vi "LVClass_Camera asynchroneImageReady.vi"(0 "Camera in":refnum<class "Camera.lvclass">, 11 "error in (no error)":errorcluster) -> (4 "Camera out":refnum<class "Camera.lvclass">, 6 "ready":bool, 15 "error out":errorcluster)   [LabVIEW 2020, in "Camera.lvclass"]
doc: "Indicates if a new image is available.\n\n<B>CameraIn</B> : Camera object.\n<B>CameraOut</B> : Camera object.\n<B>is_ready</B> : image availability in asynchronous image synchronization mode."
uses:
  Camera.lvclass
  Camera.lvclass/Camera.ctl
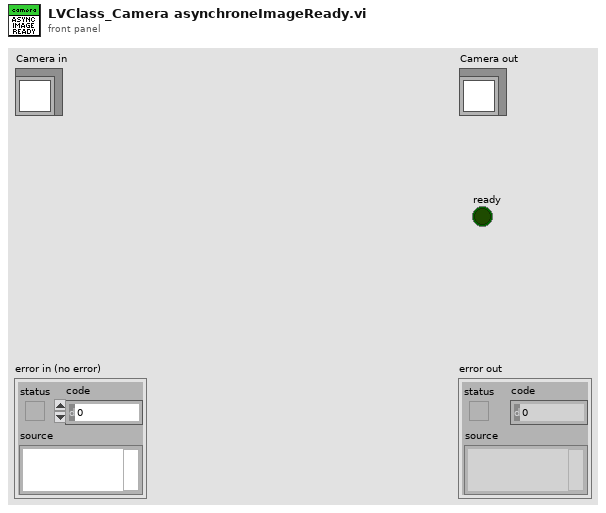
[diagram p1: front panel]
types:
  T1 = typedef "ClassID.ctl" = i64
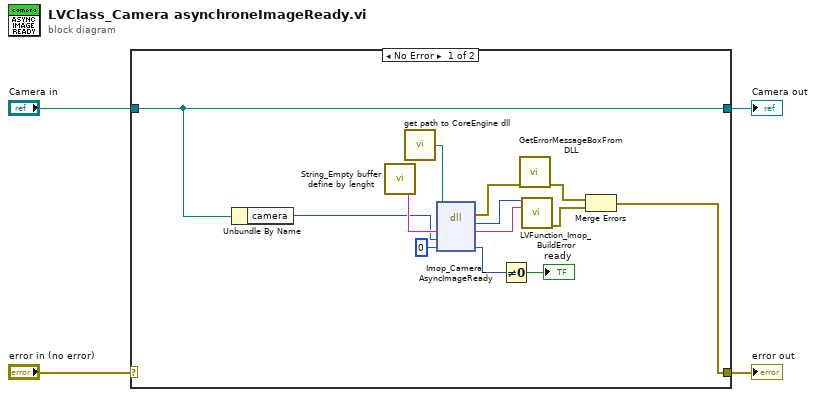
[diagram p0: block diagram]
diagram:
  n1 = case shown="No Error" "error in (no error)" {
    selector: "error in (no error)" -> [_ w19]
    tunnel: [w5 w19] -> w3
    tunnel: [w9 w18] -> w1
    tunnel: "Camera in" -> [w9 w18]
    frame No Error {
      n2 = Unbundle By Name(w9) -> ("camera"=w8:T1)
      n3 = call "String_Empty buffer define by lenght.vi"() -> ("Empty buffer"=w17:string)  [unwired: 1 in]
      n4 = call "get path to CoreEngine dll.vi"() -> ("path to c_interface_vc100.dll"=w14:path)  [unwired: 12 in, 3 out]
      n5 = dll-call lib="D:/SOFTware/HASO_v3/SVN_trunk/ImOpCoreEngine4_LV2011/DLLs/ImopEngine4_vc100.dll" fn="Imop_Camera_AsyncImageReady"(path in=w14, "message"=w17, "camera"=w8, "ready"=u8 0) -> (error out=w13:errorcluster, "return type"=w16:i32, "message"=w15:string, "ready"=w11:u8)  [unwired: 3 in, 1 out]
      n6 = Not Equal To 0?(x=w11) -> (x != 0?=→"ready":bool)
      n7 = call "GetErrorMessageBoxFromDLL.vi"("error IN"=w13) -> ("error OUT"=w7:errorcluster)  [unwired: 10 in]
      n8 = call "LVFunction_Imop_BuildError.vi"("code"=w16, "String to Prepend to source (\"\")"=w15) -> ("error out"=w6:errorcluster)  [unwired: 13 in]
      n9 = Merge Errors(w7, w6) -> (w5:errorcluster)
    }
    frame Error {
    }
  }
  "error out" <- w3
  "Camera out" <- w1
